vi "Check Class Status.vi"(11 "Scaffold Project Refs":T1) -> (3 "Is ByRef Class?":bool)   [LabVIEW 2018]
uses:
  <resource>/Framework/Providers/LVClassByRef/Scaffold Project Refs.ctl
  <resource>/Framework/Providers/LVClassByRef/LVClassByRef.lvlib
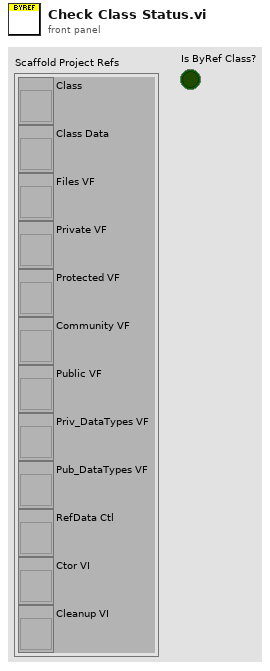
[diagram p1: front panel]
types:
  T1 = typedef "LVClassByRef.lvlib/Scaffold Project Refs.ctl" = cluster{"Class":refnum<vi>, "Class Data":refnum<vi>, "Files VF":refnum<vi>, "Private VF":refnum<vi>, "Protected VF":refnum<vi>, "Community VF":refnum<vi>, "Public VF":refnum<vi>, "Priv_DataTypes VF":refnum<vi>, "Pub_DataTypes VF":refnum<vi>, "RefData Ctl":refnum<vi>, "Ctor VI":refnum<vi>, "Cleanup VI":refnum<vi>}
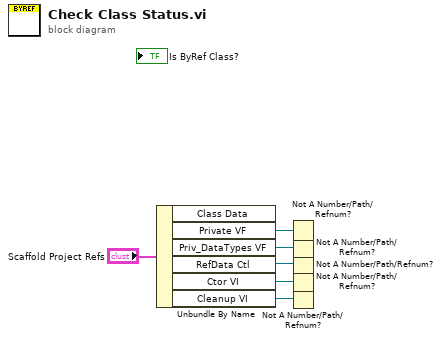
[diagram p0: block diagram]
diagram:
  n1 = Unbundle By Name("Scaffold Project Refs") -> ("Private VF"=w5:refnum<vi>, "Priv_DataTypes VF"=w1:refnum<vi>, "RefData Ctl"=w2:refnum<vi>, "Ctor VI"=w3:refnum<vi>, "Cleanup VI"=w4:refnum<vi>)  [unwired: 1 out]
  n2 = Not A Number/Path/Refnum?(number/path/refnum=w5) -> ()  [unwired: 1 out]
  n3 = Not A Number/Path/Refnum?(number/path/refnum=w1) -> ()  [unwired: 1 out]
  n4 = Not A Number/Path/Refnum?(number/path/refnum=w2) -> ()  [unwired: 1 out]
  n5 = Not A Number/Path/Refnum?(number/path/refnum=w3) -> ()  [unwired: 1 out]
  n6 = Not A Number/Path/Refnum?(number/path/refnum=w4) -> ()  [unwired: 1 out]
